vi "Variant.vi"() -> ()   [LabVIEW 2011]
panel:
  out "Recoverd string":string[](array[string])
  out "Flatened String":string[](array[string])
  out "appended array":variant[](array[variant])
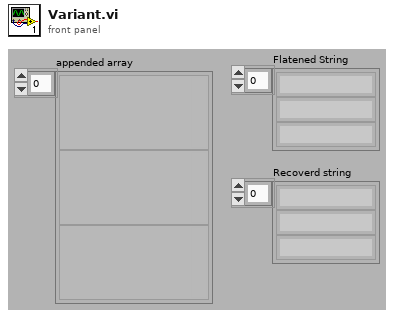
[diagram p1: front panel]
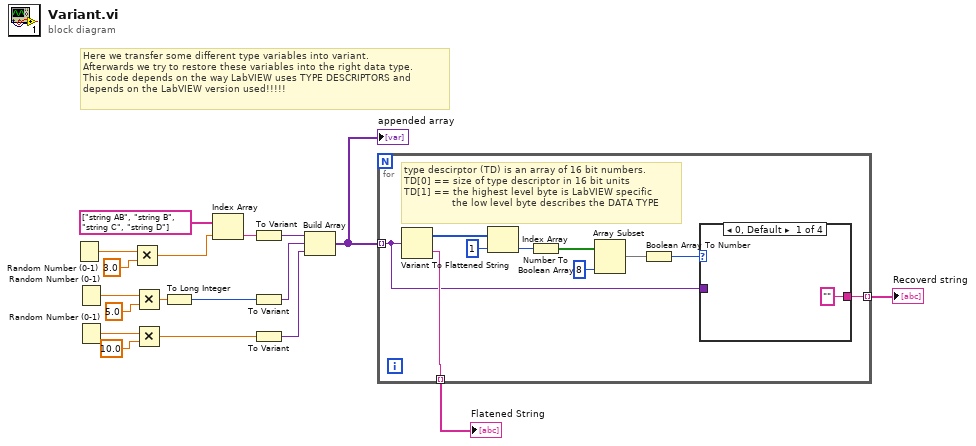
[diagram p0: block diagram]
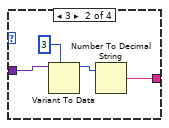
[diagram p2: hidden frame]
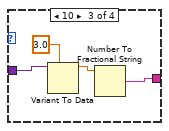
[diagram p3: hidden frame]
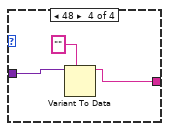
[diagram p4: hidden frame]
diagram:
  # "Here we transfer some different type variables into variant.\nAfterwards we try to restore these variables into the right data type.\nThis code depends on the way LabVIEW uses TYPE DESCRIPTORS and\ndepends on the LabVIEW version used!!!!!"
  n1 = Random Number (0-1)() -> (number: 0 to 1=w9:dbl)
  n2 = Random Number (0-1)() -> (number: 0 to 1=w16:dbl)
  n3 = Random Number (0-1)() -> (number: 0 to 1=w13:dbl)
  n4 = Multiply(x=w9, y=3.0) -> (x*y=w6:dbl)
  n5 = Multiply(x=w16, y=5.0) -> (x*y=w11:dbl)
  n6 = Multiply(x=w13, y=10.0) -> (x*y=w12:dbl)
  n7 = To Long Integer(number=w11) -> (32bit integer=w10:i32)
  n8 = Index Array(array=string[] ["string AB", "string B", "string C", "string D"] ("names"), index=w6) -> (element=w5:string)
  n9 = To Variant(anything=w5) -> (Variant=w18:variant)
  n10 = To Variant(anything=w10) -> (Variant=w17:variant)
  n11 = To Variant(anything=w12) -> (Variant=w4:variant)
  n12 = Build Array(w18, w17, w4) -> (w3:variant[])
  "appended array" <- w3
  n13 = for {
    tunnel: w3 -> [w20] mode=indexing
    tunnel: [w21] -> w2 mode=indexing
    tunnel: [w19] -> w1 mode=indexing
    # "type descirptor (TD) is an array of 16 bit numbers.\nTD[0] == size of type descriptor in 16 bit units\nTD[1] == the highest level byte is LabVIEW specific\n                the low level byte describes the DATA TYPE"
    n14 = Variant To Flattened String(Variant=w20) -> (data string=w21:string, 1:w28:i16[])
    n15 = Index Array(array=w28, index=1) -> (element=w26:i16)
    n16 = Number To Boolean Array(number=w26) -> (Boolean array=w25:bool[])
    n17 = Array Subset(array=w25, length=8) -> (w23:bool[])  [unwired: 1 in]
    n18 = Boolean Array To Number(Boolean array=w23) -> (number=w22:u32)
    n19 = case shown="0, Default" w22 {
      tunnel: w20 -> [_ w32 w37 w40]
      tunnel: ["" w30 w34 w38] -> w19
      frame 0, Default {
      }
      frame 3 {
        n20 = Variant To Data(type=3 ("y"), Variant=w32) -> (data=w31:i32)  [unwired: 1 in, 1 out]
        n21 = Number To Decimal String(number=w31) -> (decimal integer string=w30:string)  [unwired: 1 in]
      }
      frame 10 {
        n22 = Variant To Data(type=3.0 ("y"), Variant=w37) -> (data=w35:dbl)  [unwired: 1 in, 1 out]
        n23 = Number To Fractional String(number=w35) -> (F-format string=w34:string)  [unwired: 3 in]
      }
      frame 48 {
        n24 = Variant To Data(type="", Variant=w40) -> (data=w38:string)  [unwired: 1 in, 1 out]
      }
    }
  }
  "Flatened String" <- w2
  "Recoverd string" <- w1
